vi "保存方式.vi"(10 "名称或相对路径":string) -> (3 "添加的路径":path)   [LabVIEW 2014]
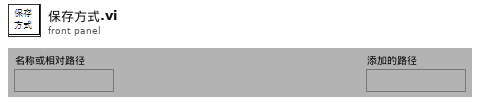
[diagram p1: front panel]
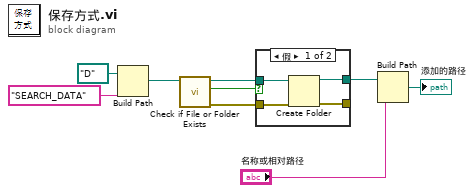
[diagram p0: block diagram]
diagram:
  n1 = Build Path(base path=path "D:/" ("基路径"), name or relative path="SEARCH_DATA" ("名称或相对路径")) -> (appended path=w7:path)
  n2 = call <vilib>:"Check if File or Folder Exists.vi"("path"=w7) -> ("error out"=w4:errorcluster, "file or folder exists?"=w6:bool, "dup path"=w5:path)  [unwired: 8 in]
  n3 = case shown="假" w6 {
    tunnel: w5 -> [w12 w15]
    tunnel: w4 -> [w13 w14]
    tunnel: [w11 w15] -> w3
    tunnel: [w10 w14] -> _
    frame False {
      n4 = Create Folder(path (use dialog)=w12, error in=w13) -> (created path=w11:path, error out=w10:errorcluster)  [unwired: 1 in, 1 out]
    }
    frame True {
    }
  }
  n5 = Build Path(base path=w3, name or relative path="名称或相对路径") -> (appended path=→"添加的路径":path)
